vi "Unpack Message.vi"(8 "error in (no error)":errorcluster, 9 "Packed Message":string, 10 "Message Name":string, 11 "Message Response in":refnum<class "Message Response.lvclass">) -> (0 "error out":errorcluster, 2 "Valid":bool, 3 "Message Response out":refnum<class "Message Response.lvclass">)   [LabVIEW 2016, in "WebSocket Networking.lvlib" / "Message Response.lvclass"]
uses:
  <userlib>/Common Components/WebSocket Networking/Message Response/Message Response.lvclass
  C:/Program Files (x86)/National Instruments/LabVIEW 2016/user.lib/Composed Systems/Stream/Mediator/Classes/Message Interface/Message Interface.lvclass
  <userlib>/Common Components/Common/command-data.ctl
  <userlib>/Common Components/WebSocket Networking/Message Response/Message Response.lvclass/Message Response.ctl
  <userlib>/Composed Systems/Stream/Mediator/Classes/Message Interface/Message Interface.lvclass
  <vilib>/addons/_JKI.lib/Serialization/JSON/JKI JSON Serialization.lvlib
  <userlib>/Common Components/Common/Common.lvlib
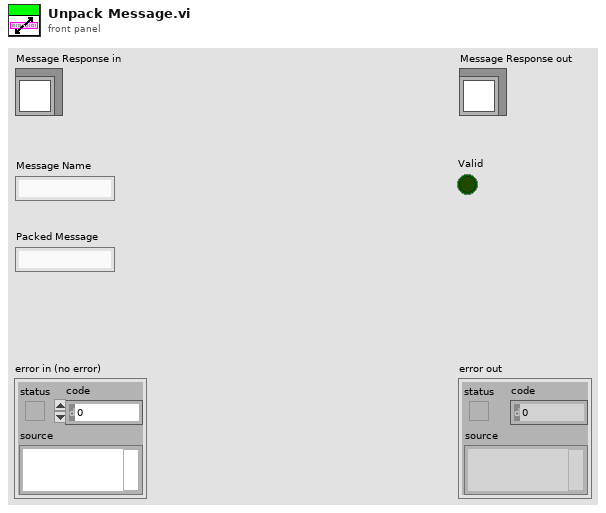
[diagram p1: front panel]
types:
  T1 = typedef "Common.lvlib/command-data.ctl" = cluster{"command":string, "data":string}
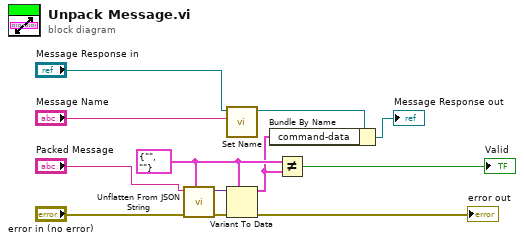
[diagram p0: block diagram]
diagram:
  w3 = T1 {"command"="", "data"=""} ("Cluster")
  n1 = call <vilib>:"Unflatten From JSON String.vi"("Type and Defaults"=w3, "error in (no error)"="error in (no error)", "JSON String"="Packed Message") -> ("error out"=w10:errorcluster, "Variant"=w11:variant)  [unwired: 7 in]
  n2 = call <userlib>:"Set Name.vi"("Name"="Message Name", "Message Interface in"="Message Response in") -> ("Message Interface out"=w12:refnum<class "Message Response.lvclass">)  [unwired: 8 in, 1 out]
  n3 = Variant To Data(error in=w10, type=w3, Variant=w11) -> (data=w2:T1, error out=→"error out":errorcluster)
  n4 = Bundle By Name(cluster=w12, "command-data"=w2) -> (→"Message Response out":refnum<class "Message Response.lvclass">)
  n5 = Not Equal?(x=w3, y=w2) -> (x != y?=→"Valid":bool)
